vi "SetChangeVariableSampleTrigger.vi"(0 "controller in":refnum<k24>, 5 "variable":string, 7 "task":i32, 11 "error in (no error)":errorcluster, 12 "trigger":i32(ring)=1 items=["OnAnyChange"=1, "OnIncrease"=2, "OnDecrease"=3]) -> (4 "controller out":refnum<k24>, 15 "error out":errorcluster)   [LabVIEW 2021]
uses:
  C:/Program Files (x86)/Aerotech/A3200/LabVIEW/2010/Bin/Aerotech.A3200.dll
  Bin/Aerotech.A3200.dll
  C:/Program Files (x86)/Aerotech/A3200/LabVIEW/2010/Bin/Aerotech.A3200.LabVIEW.dll
  Bin/Aerotech.A3200.LabVIEW.dll
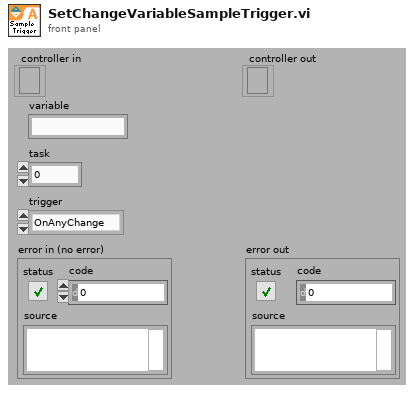
[diagram p1: front panel]
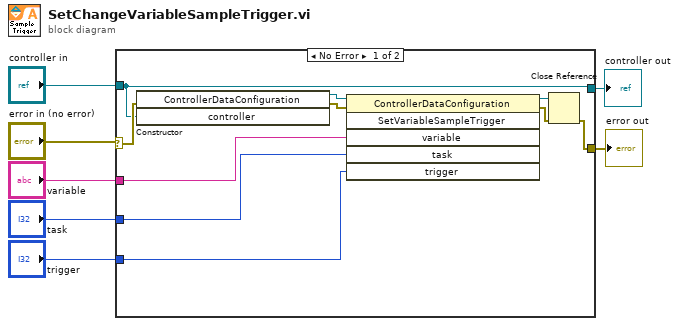
[diagram p0: block diagram]
diagram:
  n1 = case shown="No Error" "error in (no error)" {
    selector: "error in (no error)" -> [w17 w19]
    tunnel: "controller in" -> [w14 w18]
    tunnel: [w11 w19] -> w4
    tunnel: [w14 w18] -> w5
    tunnel: "trigger" -> [w8 _]
    tunnel: "task" -> [w10 _]
    tunnel: "variable" -> [w9 _]
    frame No Error {
      n2 = constructor class="ControllerDataConfiguration"(error in=w17, "controller"=w14) -> (reference out=w16:refnum<k24>, error out=w15:errorcluster)  [unwired: 2 in, 2 out]
      n3 = invoke class="ControllerDataConfiguration" method="SetVariableSampleTrigger"(reference=w16, error in=w15, "variable"=w9, "task"=w10, "trigger"=w8) -> (reference out=w12:refnum<k24>, error out=w13:errorcluster)  [unwired: 1 in, 4 out]
      n4 = Close Reference(reference=w12, error in (no error)=w13) -> (error out=w11:errorcluster)
    }
    frame Error {
    }
  }
  "controller out" <- w5
  "error out" <- w4
